vi "Move_Until_Discard.vi"(8 "error in (no error)":errorcluster, 10 "Desired Height":dbl=150.0 format="%#_13g", 11 "VISA Refnum in":refnum<visa-resource-name>="COM6") -> (0 "error out":errorcluster, 3 "VISA Refnum out":refnum<visa-resource-name>)   [LabVIEW 2018]
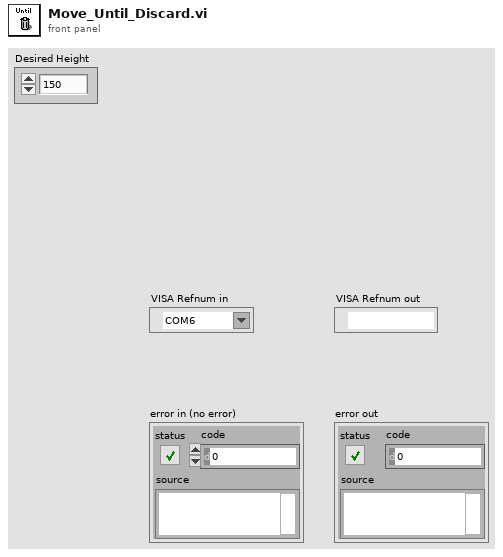
[diagram p1: front panel]
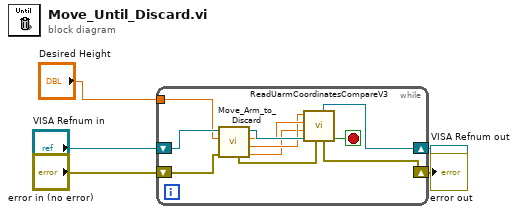
[diagram p0: block diagram]
diagram:
  n1 = while {
    shift-right: [w16] -> w4
    shift-left: "VISA Refnum in" -> [w13]
    shift-right: [w15] -> w5
    shift-left: "error in (no error)" -> [w12]
    tunnel: "Desired Height" -> [w8]
    stop <- w14 stop-if-true
    n2 = call "Move_Arm_to_Discard.vi"("Machine In"=w13, "Desired Height"=w8, "error in"=w12) -> ("error out"=w6:errorcluster, "Machine Out"=w11:refnum<visa-resource-name>, "X Coordinate"=w10:dbl, "Y Coordinate"=w9:dbl, "Z Coordinate"=w7:dbl)  [unwired: 3 in]
    n3 = call "ReadUarmCoordinatesCompareV3.vi"("error in"=w6, "Machine In"=w11, "INPUT Z Coord"=w7, "INPUT X Coord"=w10, "INPUT Y Coord"=w9) -> ("x = y?"=w14:bool, "error out"=w15:errorcluster, "Machine Out"=w16:refnum<visa-resource-name>)  [unwired: 1 in, 3 out]
  }
  "error out" <- w5
  "VISA Refnum out" <- w4
